vi "MWS Tanks.vi"(8 "Set state:":bool, 9 "Tank height":dbl, 11 "Status Message":string) -> (0 "Set":bool)   [LabVIEW 2011]
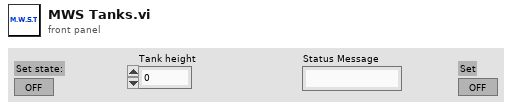
[diagram p1: front panel]
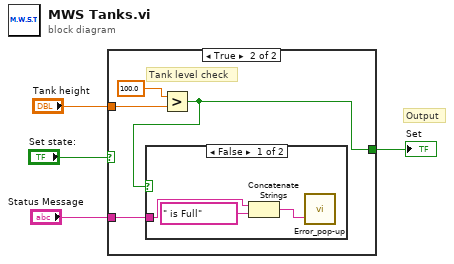
[diagram p0: block diagram]
diagram:
  # "Output"
  n1 = case shown="True" "Set state:" {
    selector: "Set state:" -> [w5 _]
    tunnel: "Tank height" -> [_ w8]
    tunnel: [w5 w6] -> w1
    tunnel: "Status Message" -> [_ w7]
    frame False {
    }
    frame True {
      # "Tank level check"
      n2 = Greater?(x=100.0, y=w8) -> (0:w6:bool)
      n3 = case shown="False" w6 {
        tunnel: w7 -> [w10 _]
        frame False {
          n4 = Concatenate Strings(w10, " is Full") -> (w11:string)
          n5 = call "Error_pop-up.vi"("New msg"=w11) -> ()  [unwired: 2 in]
        }
        frame True {
        }
      }
    }
  }
  "Set" <- w1
